vi "Ensure Unique Entries 1D Array.vi"(4 "1D Array":string[](array[string])) -> (1 "ID Array with Unique Entries":string[](array[string]))   [LabVIEW 2010]
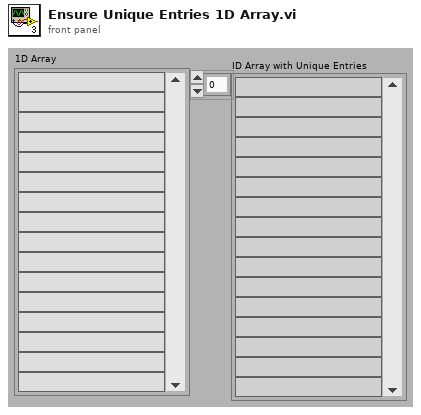
[diagram p1: front panel]
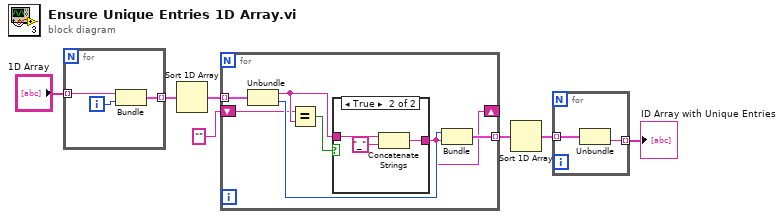
[diagram p0: block diagram]
diagram:
  n1 = for {
    tunnel: "1D Array" -> [w10] mode=indexing
    tunnel: [w8] -> w6 mode=indexing
    i -> [w9]
    n2 = Bundle("String"=w10, w9) -> (w8:cluster{"String":string, i32})  [unwired: 1 in]
  }
  n3 = Sort 1D Array(array=w6) -> (sorted array=w5:cluster{"String":string, i32}[])
  n4 = for {
    tunnel: w5 -> [w17] mode=indexing
    shift-right: [w11] -> _
    shift-left: "" ("String") -> [w12]
    tunnel: [w14] -> w3 mode=indexing
    n5 = Unbundle(w17) -> ("String"=w13:string, w15:i32)
    n6 = Equal?(x=w12, y=w13) -> (x = y?=w16:bool)
    n7 = case shown="True" w16 {
      tunnel: w13 -> [w18 w21]
      tunnel: [w18 w20] -> w11
      frame False {
      }
      frame True {
        n8 = Concatenate Strings(w21, "_" ("string")) -> (w20:string)
      }
    }
    n9 = Bundle(w15, "String"=w11) -> (w14:cluster{i32, "String":string})  [unwired: 1 in]
  }
  n10 = Sort 1D Array(array=w3) -> (sorted array=w2:cluster{i32, "String":string}[])
  n11 = for {
    tunnel: w2 -> [w23] mode=indexing
    tunnel: [w22] -> w1 mode=indexing
    n12 = Unbundle(w23) -> ("String"=w22:string)  [unwired: 1 out]
  }
  "ID Array with Unique Entries" <- w1
